vi "set cal on PDW.vi"(8 "error in (no error)":errorcluster, 10 "PDWs on channels":cluster{T1[]}[](array[cluster]), 11 "device_type in":refnum<class "device_type.lvclass">) -> (0 "error out":errorcluster, 2 "PDWs on channels":cluster{T1[]}[](array[cluster]), 3 "device_type out":refnum<class "device_type.lvclass">)   [LabVIEW 2021, in "device_type.lvclass"]
uses:
  device_type.lvclass
  pulse_tx_vis/CTL/PDW_lv2.ctl
  pulse_tx_vis/CTL/mode_type.ctl
  device_type.lvclass/device_type.ctl
  <vilib>/Analysis/coordinate.llb/Angle Units.ctl
  <vilib>/Analysis/coordinate.llb/Wrap Angle (scalar).vi
  <vilib>/Analysis/NI_AAL_Angle.lvlib
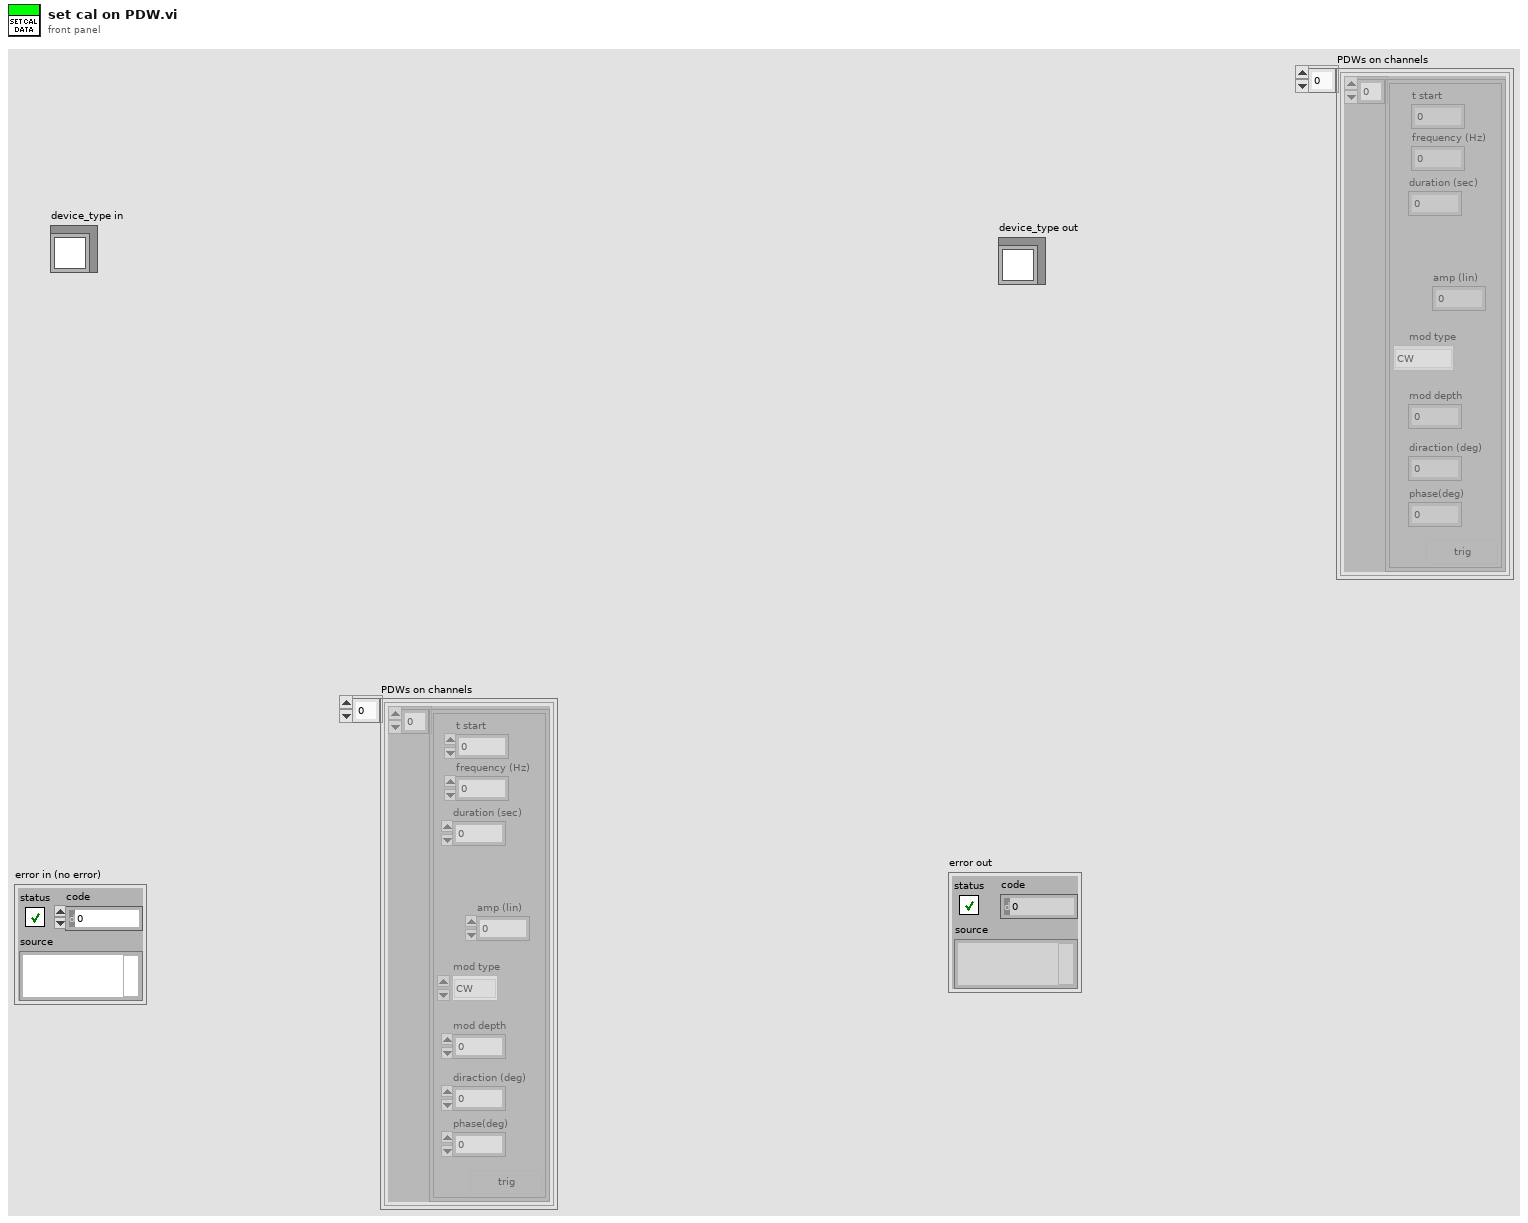
[diagram p1: front panel]
types:
  T1 = typedef "PDW_lv2.ctl" = cluster{"t start":dbl, "frequency (Hz)":dbl, "duration (sec)":dbl, "mod type":T2, "mod depth":dbl, "trig":bool, "amp (lin)":dbl, "diraction (deg)":dbl, "phase(deg)":dbl}
  T2 = typedef "mode_type.ctl" = enum8{"CW", "from memory 1", "NC - cw", "LFM", "BPSK", "QPSK"}
  T3 = cluster{"freqency":dbl[], "phase":dbl[], "amp":dbl[]}[]
  T4 = typedef "NI_AAL_Angle.lvlib/Angle Units.ctl" = i32
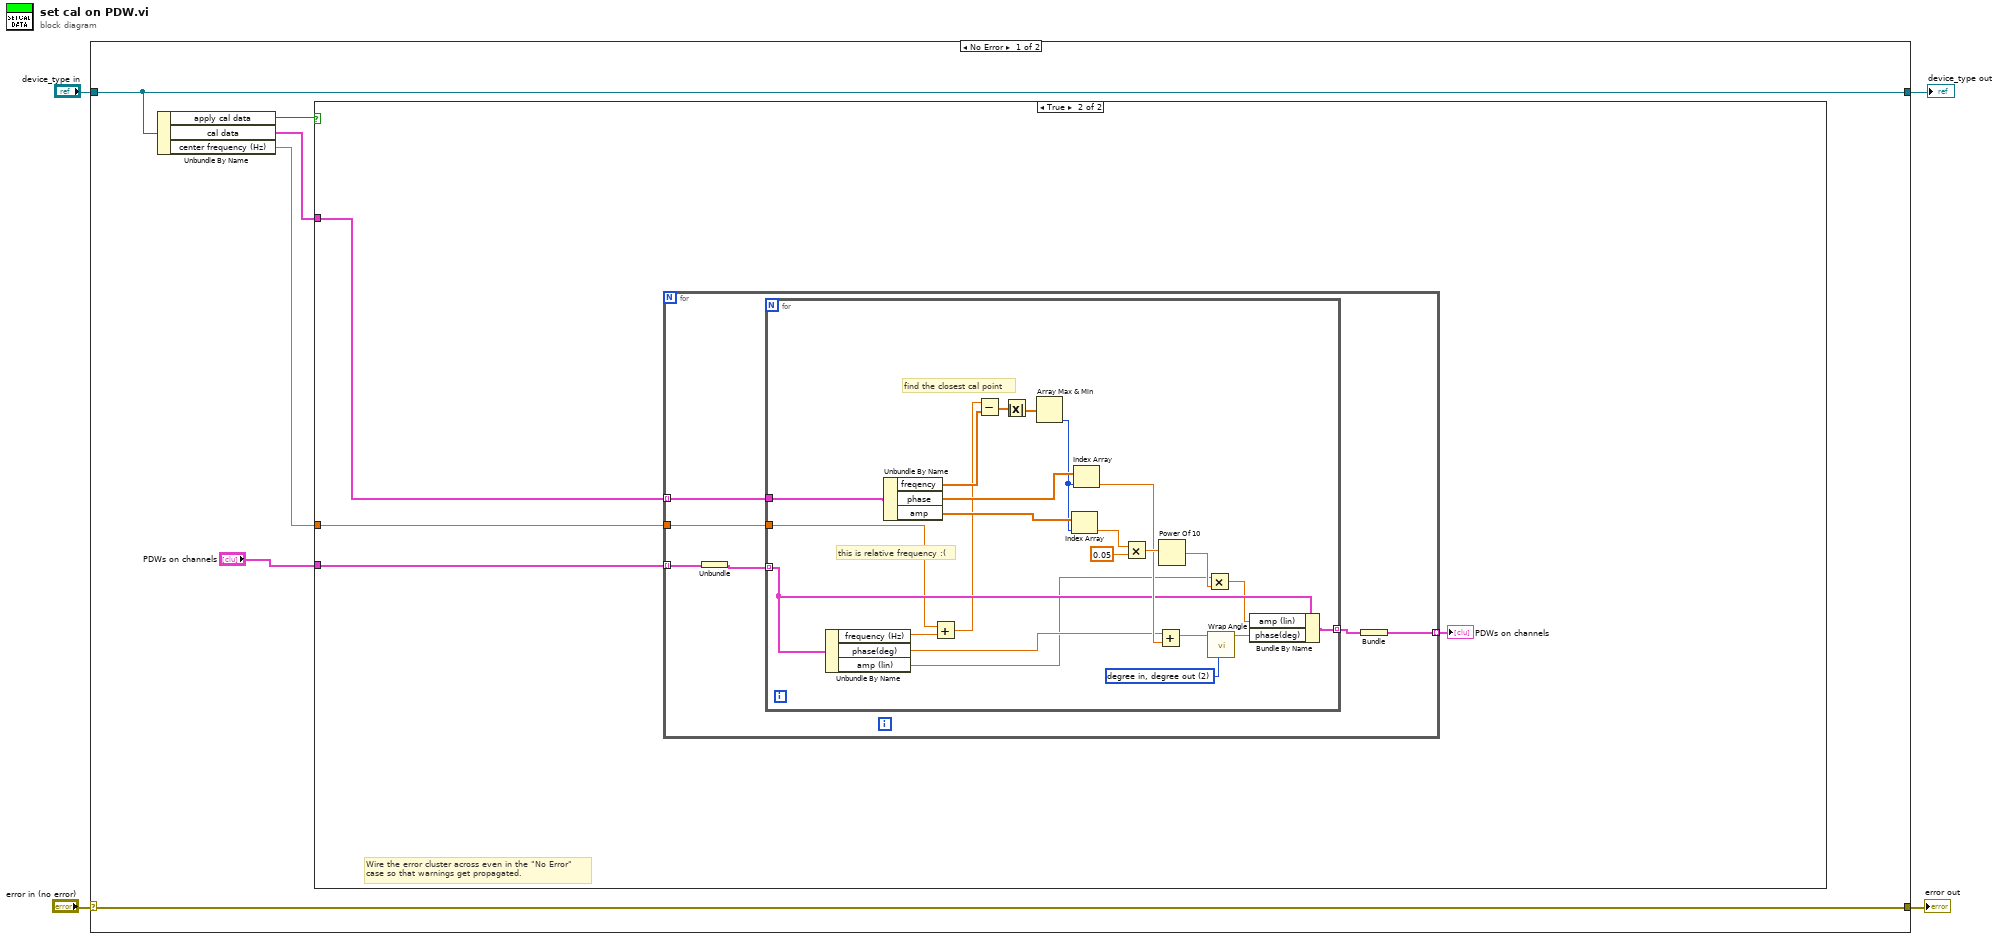
[diagram p0: block diagram]
diagram:
  n1 = case shown="No Error" "error in (no error)" {
    selector: "error in (no error)" -> [w10 w45]
    tunnel: [w10 w45] -> w3
    tunnel: [w9 w44] -> w1
    tunnel: "device_type in" -> [w9 w44]
    frame No Error {
      n2 = Unbundle By Name(w9) -> ("apply cal data"=w8:bool, "cal data"=w7:T3, "center frequency (Hz)"=w5:dbl)
      n3 = case shown="True" w8 {
        tunnel: w7 -> [_ w14]
        tunnel: "PDWs on channels" -> [_ w13]
        tunnel: w5 -> [_ w12]
        frame False {
        }
        frame True {
          # "Wire the error cluster across even in the \"No Error\"\ncase so that warnings get propagated."
          n4 = for {
            tunnel: w14 -> [w20] mode=indexing
            tunnel: w13 -> [w19] mode=indexing
            tunnel: w12 -> [w17]
            tunnel: [w15] -> w11 mode=indexing
            n5 = Unbundle(w19) -> (w18:T1[])
            n6 = for {
              tunnel: w20 -> [w43]
              tunnel: w18 -> [w31] mode=indexing
              tunnel: w17 -> [w30]
              tunnel: [w25] -> w16 mode=indexing
              w24 = T4 2 items=["radian in, radian out", "radian in, degree out", "degree in, degree out", "degree in, radian out"] ("angle units")
              # "this is relative frequency :("
              # "find the closest cal point"
              n7 = Unbundle By Name(w31) -> ("frequency (Hz)"=w29:dbl, "phase(deg)"=w28:dbl, "amp (lin)"=w23:dbl)
              n8 = Unbundle By Name(w43) -> ("freqency"=w33:dbl[], "phase"=w42:dbl[], "amp"=w41:dbl[])
              n9 = Add(x=w30, y=w29) -> (x+y=w21:dbl)
              n10 = Subtract(x=w21, y=w33) -> (x-y=w35:dbl[])
              n11 = Absolute Value(x=w35) -> (abs(x)=w36:dbl[])
              n12 = Array Max & Min(array=w36) -> (min index (indices)=w34:i32)  [unwired: 3 out]
              n13 = Index Array(array=w41, index=w34) -> (element=w40:dbl)
              n14 = Index Array(array=w42, index=w34) -> (element=w32:dbl)
              n15 = Multiply(x=w40, y=0.05) -> (x*y=w38:dbl)
              n16 = Add(x=w28, y=w32) -> (x+y=w27:dbl)
              n17 = Power Of 10(x=w38) -> (10^x=w37:dbl)
              n18 = Multiply(x=w23, y=w37) -> (x*y=w22:dbl)
              n19 = call-poly <vilib>:"Wrap Angle.vi"("angle units"=w24, "angle in"=w27) -> ("angle out"=w26:dbl)  [unwired: 8 in, 1 out]
              n20 = Bundle By Name(cluster=w31, "amp (lin)"=w22, "phase(deg)"=w26) -> (w25:T1)
            }
            n21 = Bundle(w16) -> (w15:cluster{T1[]})  [unwired: 1 in]
          }
          "PDWs on channels" <- w11
        }
      }
    }
    frame Error {
    }
  }
  "error out" <- w3
  "device_type out" <- w1
